vi "GT Get Capture Offset.vi"(0 "cardNum":i16, 1 "pLoop":i32, 5 "encoder":i16, 7 "pOffset":i32, 9 "pCount":i16, 11 "error in (no error)":errorcluster caption="错误输入（无错误）") -> (3 "pLoop out":i32, 4 "function return":i16, 8 "pOffset out":i32, 10 "pCount out":i16, 15 "error out":errorcluster caption="错误输出")   [LabVIEW 2020, in "gts1.lvlib"]
doc: "GT_API GT_GetCaptureOffset(short cardNum,short encoder,long *pOffset,short *pCount,long *pLoop);"
uses:
  gts1.lvlib
  dll/32bit/multi_card/gts.dll
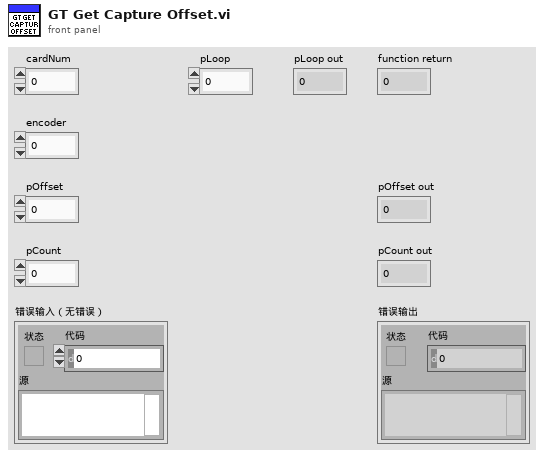
[diagram p1: front panel]
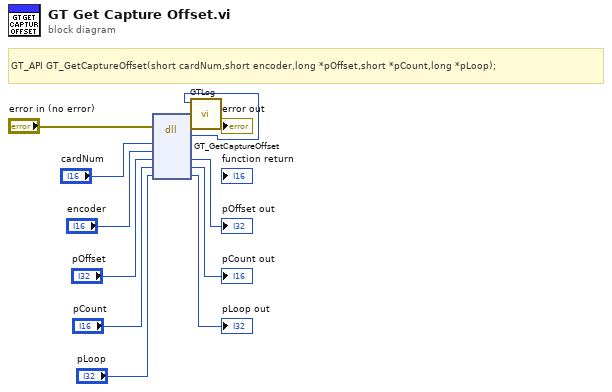
[diagram p0: block diagram]
diagram:
  # "GT_API GT_GetCaptureOffset(short cardNum,short encoder,long *pOffset,short *pCount,long *pLoop);"
  n1 = dll-call lib="C:/1228/dll/32bit/multi_card/gts.dll" fn="GT_GetCaptureOffset"(error in="error in (no error)", "cardNum"="cardNum", "encoder"="encoder", "pOffset"="pOffset", "pCount"="pCount", "pLoop"="pLoop") -> (error out=w3:errorcluster, w1:i16, "pOffset"=→"pOffset out":i32, "pCount"=→"pCount out":i16, "pLoop"=→"pLoop out":i32)  [unwired: 4 in, 1 out]
  n2 = call "GTLog.vi"("error in (no error)"=w3, "Numeric"=w1) -> ("error out"=→"error out":errorcluster)  [unwired: 9 in]
